vi "MSScript_Exe_ArrVarDef.vi"(8 "error in (no error)":errorcluster, 9 "Expression index":i32, 11 "MSScript in":refnum<class "MSScript.lvclass">) -> (0 "Error out":errorcluster, 1 "Next expression index":i32, 3 "MSScript out":refnum<class "MSScript.lvclass">)   [LabVIEW 2018, in "MSScript.lvclass"]
uses:
  MSScript.lvclass
  MSScript.lvclass/MSScript.ctl
  MSScript_Error_(6001)VariableError.vi
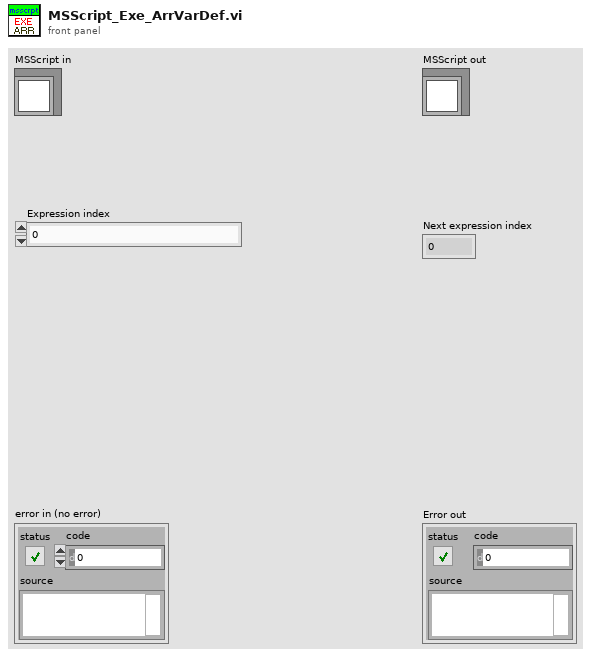
[diagram p1: front panel]
types:
  T1 = cluster{"Type":string, "NAME":cluster{"STR":string, "Start":i32}, "PARAMs":cluster{"STR":string, "Start":i32}[]}[]
  T2 = cluster{"Type":string, "NAME":cluster{"STR":string, "Start":i32}, "PARAMs":cluster{"STR":string, "Start":i32}[]}
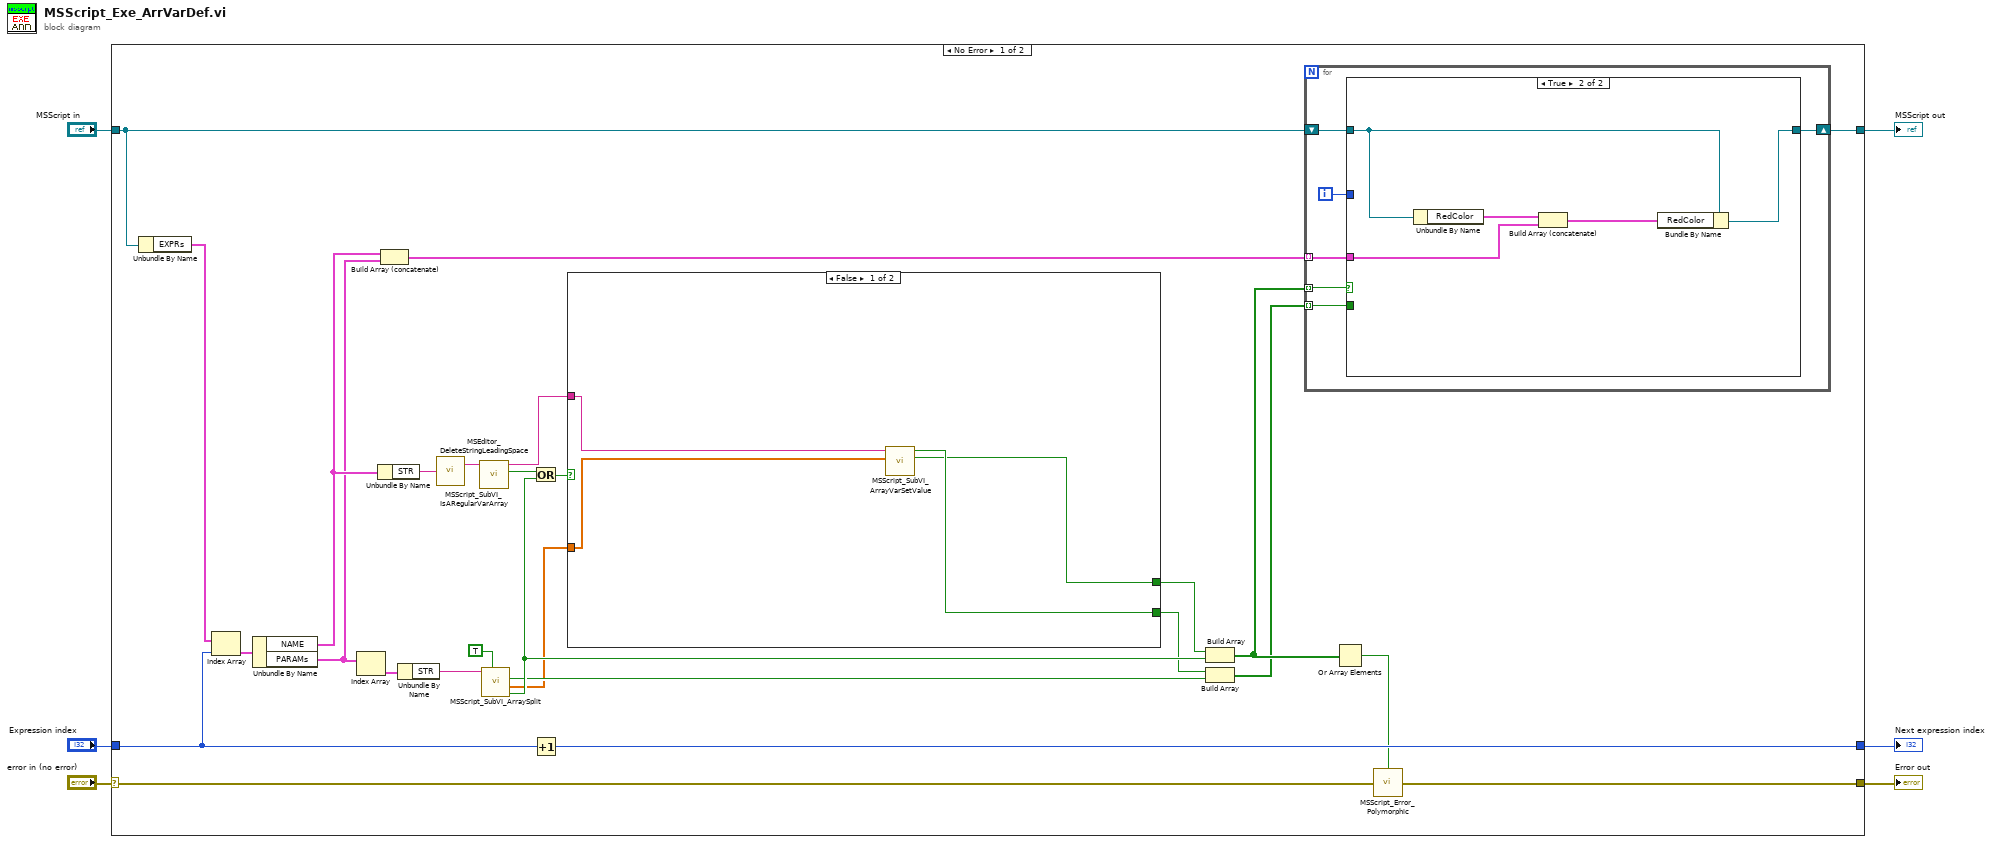
[diagram p0: block diagram]
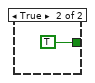
[diagram p2: hidden frame]
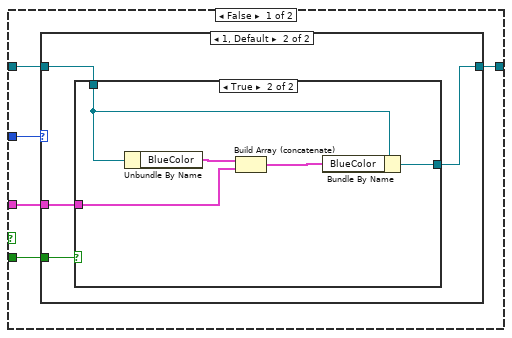
[diagram p3: hidden frame]
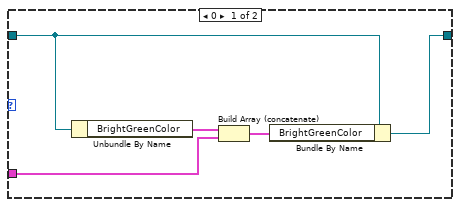
[diagram p4: hidden frame]
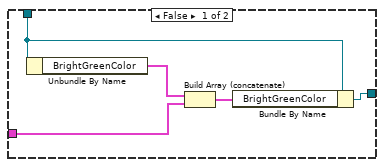
[diagram p5: hidden frame]
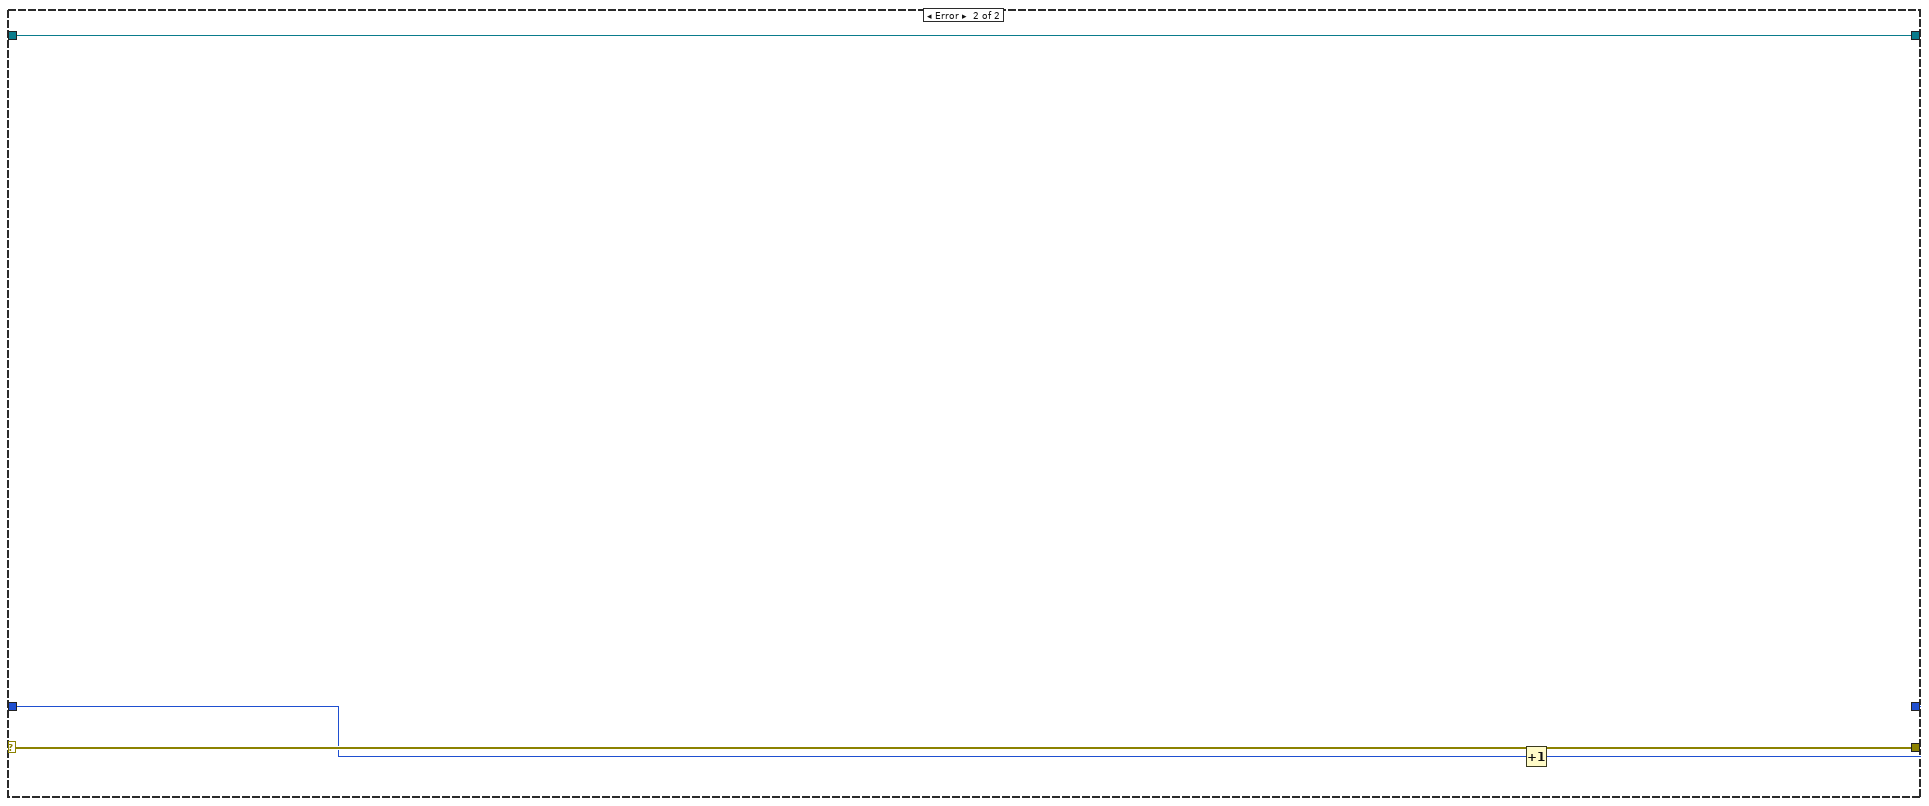
[diagram p6: hidden frame]
diagram:
  n1 = case shown="No Error" "error in (no error)" {
    selector: "error in (no error)" -> [w27 w77]
    tunnel: [w28 w75] -> w6
    tunnel: "MSScript in" -> [w21 w74]
    tunnel: "Expression index" -> [w29 w76]
    tunnel: [w26 w77] -> w2
    tunnel: [w20 w74] -> w1
    frame No Error {
      n2 = Unbundle By Name(w21) -> ("EXPRs"=w33:T1)
      n3 = Index Array(array=w33, index=w29) -> (element=w32:T2)
      n4 = Unbundle By Name(w32) -> ("NAME"=w24:cluster{"STR":string, "Start":i32}, "PARAMs"=w23:cluster{"STR":string, "Start":i32}[])
      n5 = Index Array(array=w23) -> (element=w30:cluster{"STR":string, "Start":i32})  [unwired: 1 in]
      n6 = Unbundle By Name(w24) -> ("STR"=w31:string)
      n7 = Build Array (concatenate)(w24, w23) -> (w22:cluster{"STR":string, "Start":i32}[])
      n8 = Unbundle By Name(w30) -> ("STR"=w16:string)
      n9 = call "MSEditor_DeleteStringLeadingSpace.vi"("string in"=w31) -> ("string after leading space"=w18:string)  [unwired: 1 out]
      n10 = call "MSScript_SubVI_IsARegularVarArray.vi"("VarString in"=w18) -> ("irregular"=w17:bool, "VarString out"=w10:string)  [unwired: 6 in, 1 out]
      n11 = call "MSScript_SubVI_ArraySplit.vi"("GetValue? (F)"=TRUE ("GetValue"), "VarString in"=w16) -> ("Value Error?"=w14:bool, "ArrayVariable out"=w9:ext[], "Is a variable?"=w13:bool)  [unwired: 6 in, 1 out]
      n12 = Or(x=w17, y=w14) -> (x .or. y?=w11:bool)
      n13 = Increment(x=w29) -> (x+1=w28:i32)
      n14 = case shown="False" w11 {
        tunnel: w10 -> [w37 _]
        tunnel: w9 -> [w36 _]
        tunnel: [w35 _] -> w7
        tunnel: [w34 TRUE ("Value Error?")] -> w8
        frame False {
          n15 = call "MSScript_SubVI_ArrayVarSetValue.vi"("ArrayValue in"=w36, "VarString in"=w37) -> ("Value Error?"=w34:bool, "isVar?"=w35:bool)  [unwired: 8 in]
        }
        frame True {
        }
      }
      n16 = Build Array(w8, w14) -> (w19:bool[])
      n17 = Build Array(w7, w13) -> (w15:bool[])
      n18 = for {
        tunnel: w19 -> [w42] mode=indexing
        tunnel: w22 -> [w41] mode=indexing
        shift-right: [w43] -> w20
        shift-left: w21 -> [w44]
        tunnel: w15 -> [w39] mode=indexing
        i -> [w40]
        n19 = case shown="True" w42 {
          tunnel: w44 -> [w47 w73]
          tunnel: [w48 w72] -> w43
          tunnel: w41 -> [w46 w70]
          tunnel: w40 -> [w49 _]
          tunnel: w39 -> [w45 _]
          frame False {
            n20 = case shown="1, Default" w49 {
              tunnel: [w53 w57] -> w48
              tunnel: w47 -> [w54 w58]
              tunnel: w46 -> [w51 w56]
              tunnel: w45 -> [_ w55]
              frame 0 {
                n21 = Unbundle By Name(w54) -> ("BrightGreenColor"=w52:cluster{"STR":string, "Start":i32}[])
                n22 = Build Array (concatenate)(w52, w51) -> (w50:cluster{"STR":string, "Start":i32}[])
                n23 = Bundle By Name(cluster=w54, "BrightGreenColor"=w50) -> (w53:refnum<class "MSScript.lvclass">)
              }
              frame 1, Default {
                n24 = case shown="True" w55 {
                  tunnel: w58 -> [w60 w68]
                  tunnel: [w59 w67] -> w57
                  tunnel: w56 -> [w61 w65]
                  frame False {
                    n25 = Unbundle By Name(w60) -> ("BrightGreenColor"=w63:cluster{"STR":string, "Start":i32}[])
                    n26 = Build Array (concatenate)(w63, w61) -> (w62:cluster{"STR":string, "Start":i32}[])
                    n27 = Bundle By Name(cluster=w60, "BrightGreenColor"=w62) -> (w59:refnum<class "MSScript.lvclass">)
                  }
                  frame True {
                    n28 = Unbundle By Name(w68) -> ("BlueColor"=w66:cluster{"STR":string, "Start":i32}[])
                    n29 = Build Array (concatenate)(w66, w65) -> (w64:cluster{"STR":string, "Start":i32}[])
                    n30 = Bundle By Name(cluster=w68, "BlueColor"=w64) -> (w67:refnum<class "MSScript.lvclass">)
                  }
                }
              }
            }
          }
          frame True {
            n31 = Unbundle By Name(w73) -> ("RedColor"=w71:cluster{"STR":string, "Start":i32}[])
            n32 = Build Array (concatenate)(w71, w70) -> (w69:cluster{"STR":string, "Start":i32}[])
            n33 = Bundle By Name(cluster=w73, "RedColor"=w69) -> (w72:refnum<class "MSScript.lvclass">)
          }
        }
      }
      n34 = Or Array Elements(Boolean array=w19) -> (logical OR=w25:bool)
      n35 = call-poly "MSScript_Error_Polymorphic.vi"("error in (no error)"=w27, "ErrBoolean"=w25) -> ("error out"=w26:errorcluster)
    }
    frame Error {
      n36 = Increment(x=w76) -> (x+1=w75:i32)
    }
  }
  "Next expression index" <- w6
  "Error out" <- w2
  "MSScript out" <- w1
